vi "Center Dialog on Caller.vi"(8 "error in":errorcluster, 9 "Dialog VI":refnum<vi>, 11 "Calling VI in":refnum<vi>) -> (0 "error out":errorcluster, 1 "Calling VI out":refnum<vi>)   [LabVIEW 2020]
doc: "Centers the front panel of a dialog VI in relation to the calling VI."
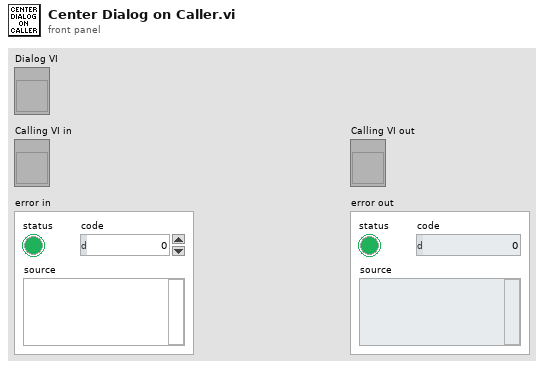
[diagram p1: front panel]
types:
  T1 = typedef "LVAllMonitorsDisplayTypeDef.ctl" = cluster{"Bounds":cluster{"Left":i16, "Top":i16, "Right":i16, "Bottom":i16}, "Depth":i16}[]
  T2 = typedef "LVRectTypeDef.ctl" = cluster{"Left":i16, "Top":i16, "Right":i16, "Bottom":i16}
  T3 = cluster{"left":i16, "top":i16, "right":i16, "bottom":i16}
  T4 = cluster{"Bounds":cluster{"Left":i16, "Top":i16, "Right":i16, "Bottom":i16}, "Depth":i16}
  T5 = cluster{"Left":i16, "Top":i16, "Right":i16, "Bottom":i16}
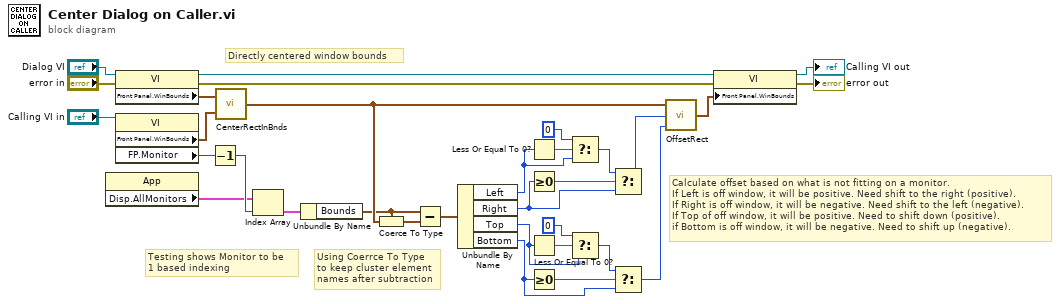
[diagram p0: block diagram]
diagram:
  # "Testing shows Monitor to be\n1 based indexing"
  # "Directly centered window bounds"
  # "Calculate offset based on what is not fitting on a monitor.\nIf Left is off window, it will be positive. Need shift to the right (positive).\nIf Right is off window, it will be negative. Need shift to the left (negative).\nIf Top of off window, it will be positive. Need to shift down (positive).\nif Bottom is off window, it will be negative. Need to shift up (negative)."
  # "Using Coerrce To Type\nto keep cluster element\nnames after subtraction"
  n1 = property class="App"() -> ("Disp.AllMonitors"=w10:T1)  [unwired: 2 in, 2 out]
  n2 = property class="VI"(reference="Dialog VI", error in="error in") -> (reference out=w5:refnum<vi>, error out=w32:errorcluster, "Front Panel.WinBounds"=w7:T2)
  n3 = property class="VI"(reference="Calling VI in") -> ("Front Panel.WinBounds"=w3:T2, "FP.Monitor"=w8:u16)  [unwired: 1 in, 2 out]
  n4 = Decrement(x=w8) -> (x-1=w11:u16)
  n5 = call <vilib>:"CenterRectInBnds.vi"("bounds"=w3, "rect"=w7) -> ("centered rect"=w29:T3)
  n6 = Index Array(array=w10, index=w11) -> (element=w9:T4)
  n7 = Unbundle By Name(w9) -> ("Bounds"=w13:T5)
  n8 = Coerce To Type(0:w29, 1:w13) -> (2:w12:T5)
  n9 = Subtract(x=w13, y=w12) -> (x-y=w14:T5)
  n10 = Unbundle By Name(w14) -> ("Left"=w2:i16, "Right"=w19:i16, "Top"=w24:i16, "Bottom"=w25:i16)
  n11 = Less Or Equal To 0?(x=w2) -> (x <= 0?=w15:bool)
  n12 = Greater Or Equal To 0?(x=w19) -> (x >= 0?=w17:bool)
  n13 = Less Or Equal To 0?(x=w24) -> (x <= 0?=w23:bool)
  n14 = Greater Or Equal To 0?(x=w25) -> (x >= 0?=w21:bool)
  n15 = Select(t=i16 0 ("Left"), s=w15, f=w2) -> (s? t:f=w18:i16)
  n16 = Select(t=i16 0 ("Left"), s=w23, f=w24) -> (s? t:f=w20:i16)
  n17 = Select(t=w18, s=w17, f=w19) -> (s? t:f=w27:i16)
  n18 = Select(t=w20, s=w21, f=w25) -> (s? t:f=w28:i16)
  n19 = call <vilib>:"OffsetRect.vi"("v"=w28, "h"=w27, "rect"=w29) -> ("offset rect"=w26:T3)
  n20 = property class="VI"(reference=w5, error in=w32, "Front Panel.WinBounds"=w26) -> (reference out=→"Calling VI out":refnum<vi>, error out=→"error out":errorcluster)
